vi "Get measurementservice_DICloseSessionResponse.vi"(8 "error in (no error)":errorcluster, 11 "gRPCid":T3) -> (0 "error out":errorcluster, 2 "Message Data":T1, 3 "gRPCid out":T3)   [LabVIEW 2019, in "ctet_dio.lvlib" / "ctet_dio.lvclass"]
uses:
  ctet_dio.lvclass
  gRPC lvSupport/Server API/typeDefs/grpcId.ctl
  measurementservice_DICloseSessionResponse_Data.ctl
  measurementservice_ErrorOut/measurementservice_ErrorOut_Data.ctl
  a51dd2a7-b5c1-4c09-9df4-8cd9d3bd0c19.vi
  gRPC lvSupport/Server API/Server/Get Server DLL Path.vi
  gRPC lvSupport/gprc-lvsupport.lvlib
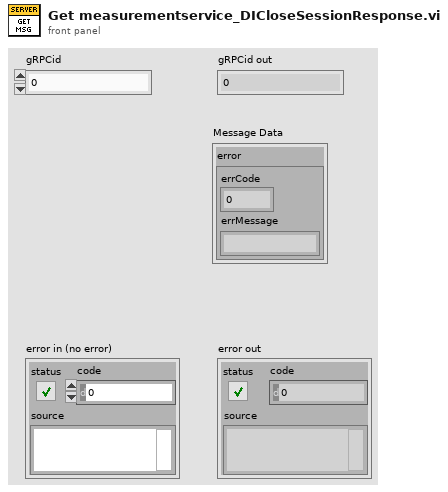
[diagram p1: front panel]
types:
  T1 = typedef "ctet_dio.lvlib/ctet_dio.lvclass/measurementservice_DICloseSessionResponse_Data.ctl" = cluster{"error":T2}
  T2 = typedef "ctet_dio.lvlib/ctet_dio.lvclass/measurementservice_ErrorOut_Data.ctl" = cluster{"errCode":i64, "errMessage":string}
  T3 = typedef "ctet_dio.lvlib/gprc-lvsupport.lvlib/grpcId.ctl" = u64
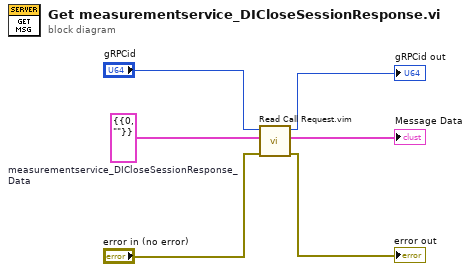
[diagram p0: block diagram]
diagram:
  w2 = T1 {"error"={"errCode"=0, "errMessage"=""}}  # measurementservice_DICloseSessionResponse_Data
  n1 = call "Read Call Request.vim"("error in (no error)"="error in (no error)", "Data Type"=w2, "gRPCid in"="gRPCid") -> ("error out"=→"error out":errorcluster, "Request Data"=→"Message Data":T1, "gRPCid out"=→"gRPCid out":T3)  [unwired: 6 in]
